vi "Set Waveform Quadrature.vi"(8 "error in (no error)":errorcluster, 10 "Quadratude":string, 11 "Waveform in":waveform(dbl)) -> (0 "error out":errorcluster, 3 "Waveform out":waveform(dbl))   [LabVIEW 2019, in "Instrument.Lockin.lvlib" / "Instrument.DAQ.lvclass"]
uses:
  Instrument.DAQ.lvclass
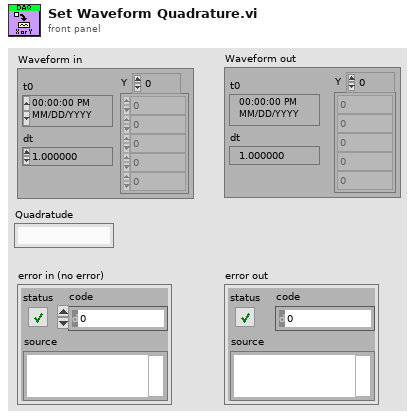
[diagram p1: front panel]
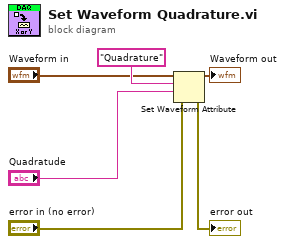
[diagram p0: block diagram]
diagram:
  n1 = Set Waveform Attribute(4:"error in (no error)", 5:"Quadratude", 6:"Quadrature" ("name"), 7:"Waveform in") -> (0:→"error out":errorcluster, 3:→"Waveform out":waveform(dbl))  [unwired: 1 out]
